vi "ALLARMI_VI.vi"(7 "simulazione":bool, 8 "error in (no error)":errorcluster, 9 "STORICO":refnum<vi>, 10 "STATO SOGLIE IMPOSTATE":refnum<vi>, 11 "Queue Name":string="ALLARMI_Q") -> (0 "error out":errorcluster, 2 "Stopped":bool)   [LabVIEW 2019]
uses:
  TypeDef/cluster allarme cost.ctl
  TypeDef/cluster allarme interp.ctl
  <vilib>/Utility/miscctls.llb/LVRowAndColumnTypeDef.ctl
  <vilib>/Utility/file.llb/Write To Spreadsheet File (string).vi
panel:
  in  "Percorso salvataggio":path
  in  "SALVA STORICO ALLARMI":bool
  out "Array soglie interpolate out":T1[](array[typedef])
  out "Array soglie costanti out":T2[](array[typedef]) caption="STORICO ALLARMI"
  out "DATA OUT":cluster{T2[], T1[]} caption="SITUAZIONE ATTUALE ALLARMI"
  out "elements in queue":i32
  out "STATO":string
  out "LOOP TIME (ms)":u32
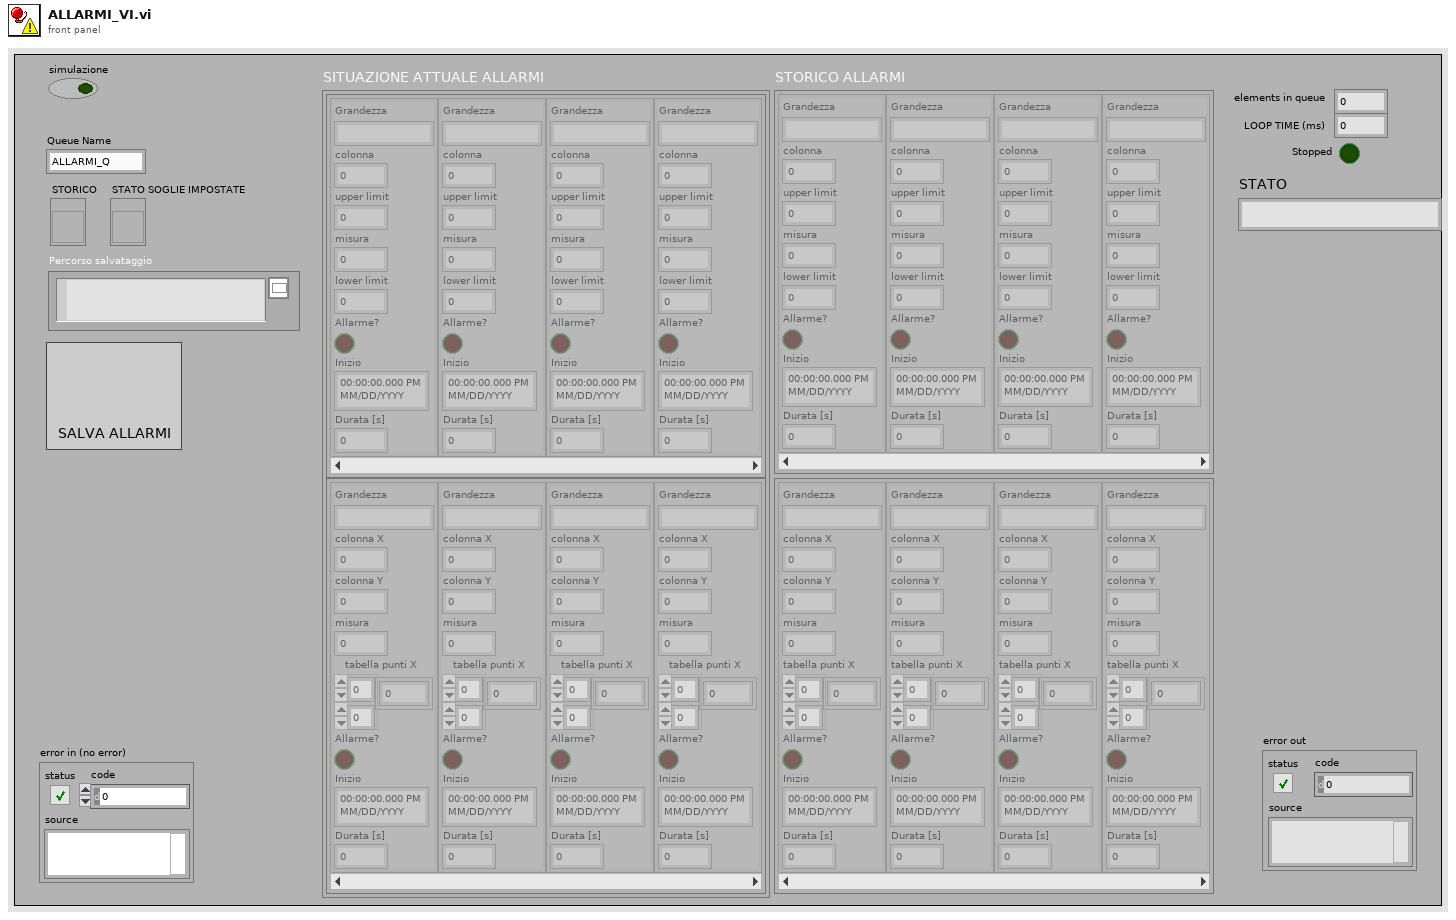
[diagram p1: front panel]
types:
  T1 = typedef "cluster allarme interp.ctl" = cluster{"Grandezza":string, "colonna X":i32, "colonna Y":i32, "misura":dbl, "tabella punti X":dbl[][], "Allarme?":bool, "Inizio":timestamp, "Durata [s]":dbl}
  T2 = typedef "cluster allarme cost.ctl" = cluster{"Grandezza":string, "colonna":i32, "upper limit":dbl, "misura":dbl, "lower limit":dbl, "Allarme?":bool, "Inizio":timestamp, "Durata [s]":dbl}
  T3 = typedef "LVRowAndColumnTypeDef.ctl" = cluster{"Row":i32, "Column":i32}
  T4 = cluster{"Array soglie costanti":T2[], "Array soglie interpolate":T1[]}
  T5 = cluster{"Array of elements":cluster{"String":string, "variant":variant}[], "Single element":cluster{"String":string, "variant":variant}, "enque at\nopposite end (F)":bool, "no replications (F)":bool}
  T6 = enum32{"Invalid", "Standard", "Closed", "Hidden", "Minimized", "Maximized"}
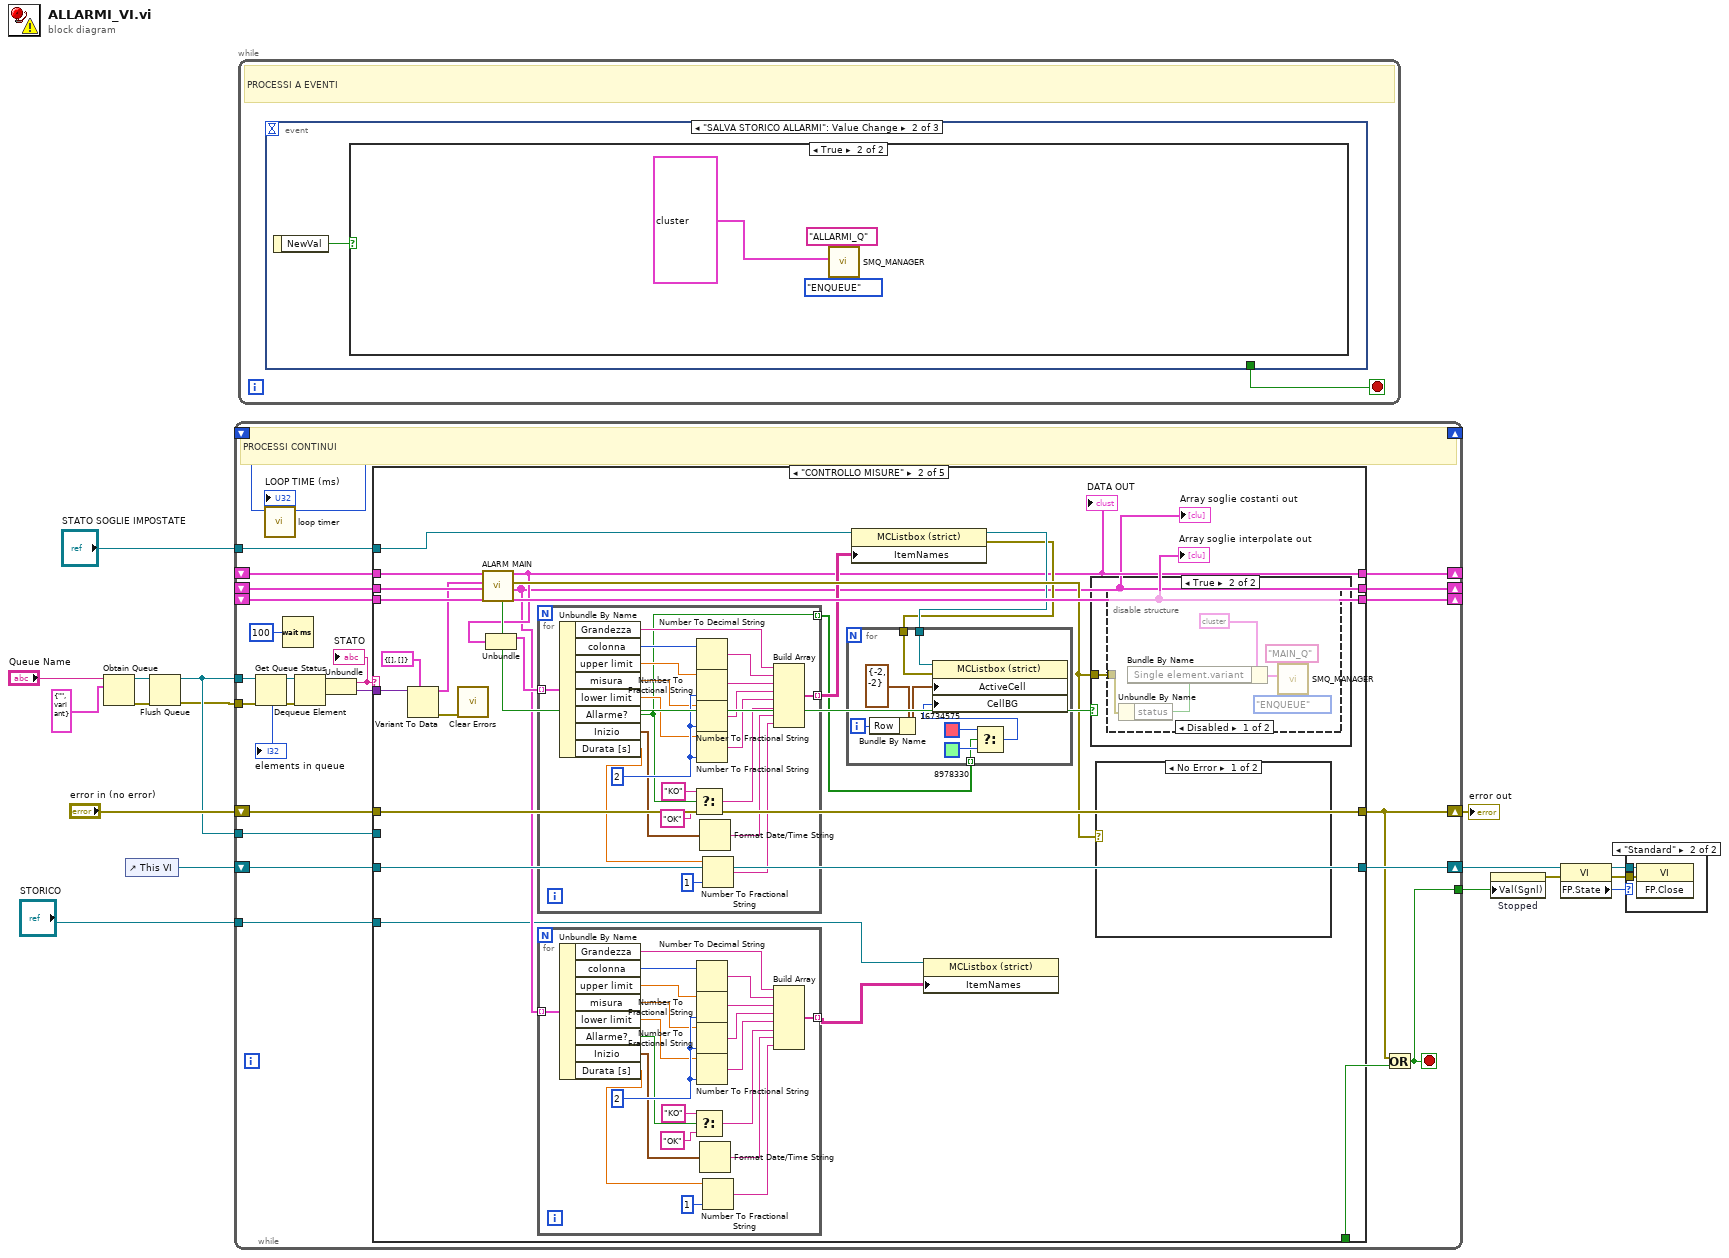
[diagram p0: block diagram]
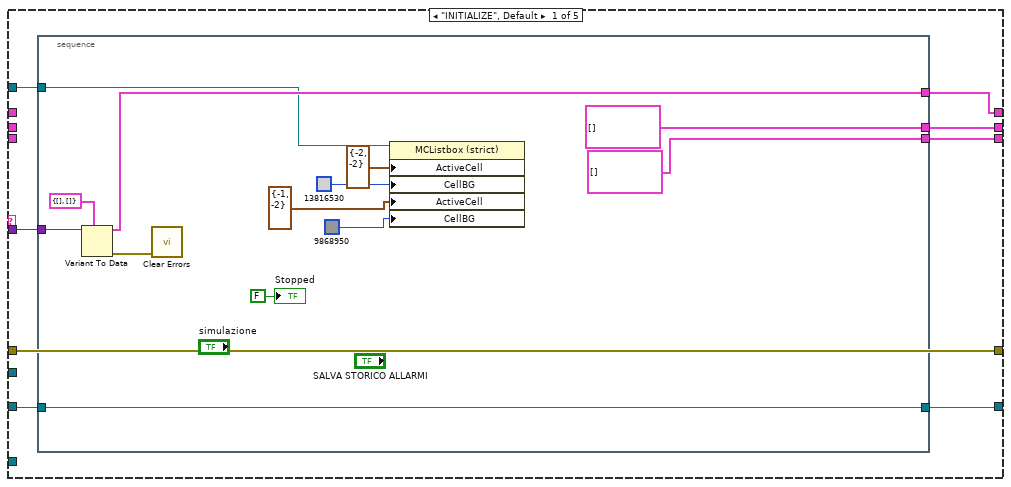
[diagram p3: hidden frame]
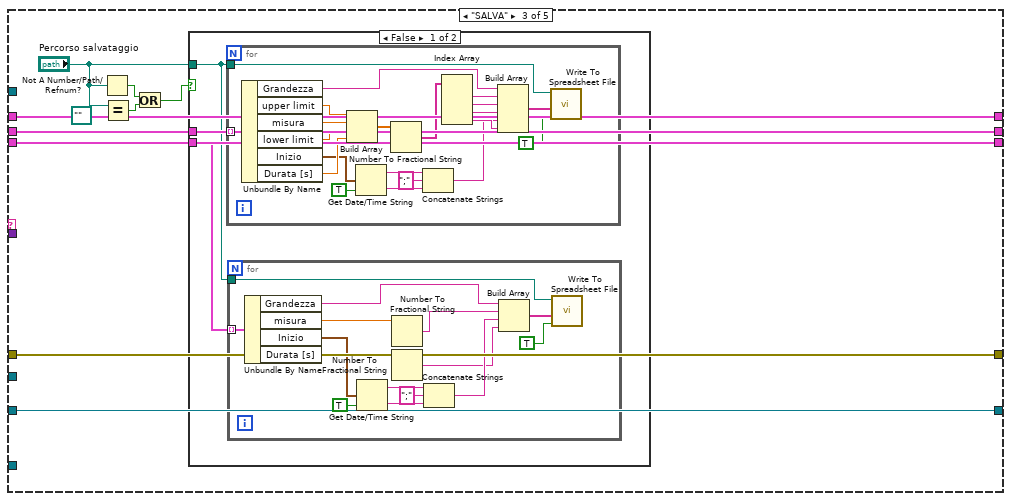
[diagram p7: hidden frame]
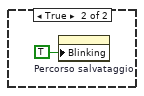
[diagram p8: hidden frame]
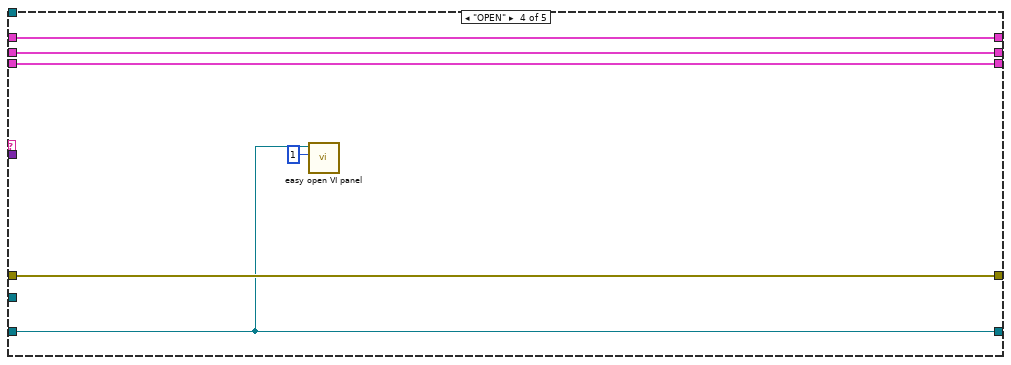
[diagram p9: hidden frame]
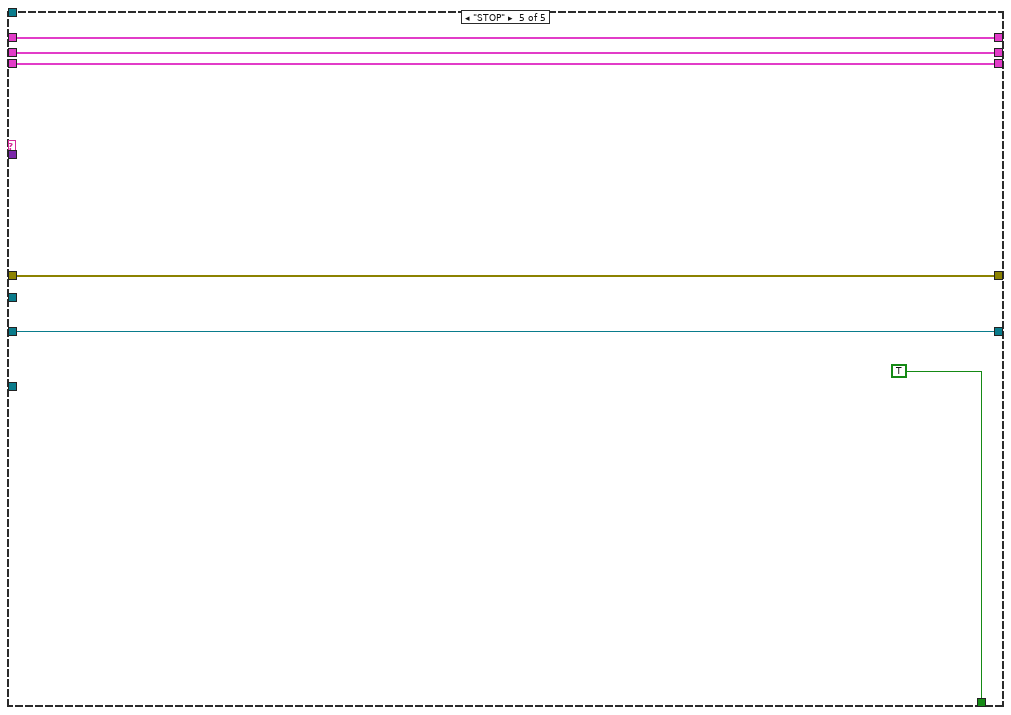
[diagram p10: hidden frame]
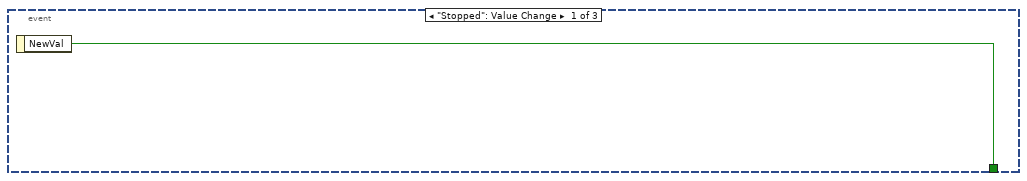
[diagram p11: hidden frame]
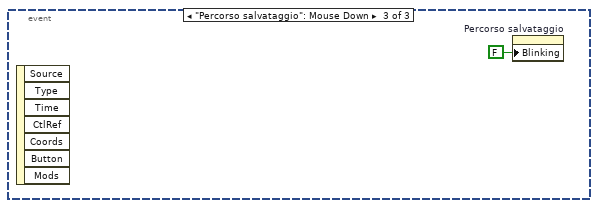
[diagram p13: hidden frame]
diagram:
  n1 = Obtain Queue(name (unnamed)="Queue Name", element data type=cluster{"String":string, "variant":variant} {"String"="", "variant"=variant} ("element")) -> (queue out=w7:refnum<queue>, error out=w6:errorcluster)  [unwired: 3 in, 1 out]
  n2 = control-ref of="This VI"() -> (w3:refnum<vi>)
  n3 = Flush Queue(queue=w7, error in (no error)=w6) -> (queue out=w5:refnum<queue>, error out=w4:errorcluster)  [unwired: 1 out]
  n4 = while {
    shift-right: [w44] -> _
    shift-left: _ -> [w43]
    shift-right: [w41] -> w10
    shift-left: w3 -> [w40]
    shift-right: [w37] -> w13
    shift-left: "error in (no error)" -> [w39]
    tunnel: w5 -> [w31]
    tunnel: w4 -> [w30]
    tunnel: [w34] -> w14
    tunnel: w5 -> [w32]
    shift-right: [w25] -> _
    shift-left: _ -> [w24]
    shift-right: [w23] -> _
    shift-left: _ -> [w22]
    shift-right: [w21] -> _
    shift-left: _ -> [w20]
    tunnel: "STATO SOGLIE IMPOSTATE" -> [w19]
    tunnel: "STORICO" -> [w18]
    stop <- w34 stop-if-true
    # "PROCESSI CONTINUI"
    n5 = Get Queue Status(queue=w31, error in (no error)=w30) -> (queue out=w28:refnum<queue>, error out=w29:errorcluster, # elements in queue=→"elements in queue":i32)  [unwired: 1 in, 5 out]
    n6 = call <userlib>:"loop timer.vi"("millisecond timer IN"=w43) -> ("millisecond timer OUT"=w44:u32, "LOOP TIME (ms)"=→"LOOP TIME (ms)":u32)  [unwired: 9 in]
    n7 = Wait (ms)(milliseconds to wait=u32 100) -> ()  [unwired: 1 out]
    n8 = Dequeue Element(queue=w28, error in (no error)=w29) -> (element=w36:cluster{"String":string, "variant":variant})  [unwired: 1 in, 3 out]
    n9 = Unbundle(w36) -> ("String"=w33:string, "variant"=w35:variant)
    "STATO" <- w33
    n10 = case shown="\"CONTROLLO MISURE\"" w33 {
      tunnel: [_ _ _ _ TRUE] -> w38
      tunnel: [w52 w87 w155 w200 w206] -> w41
      tunnel: w40 -> [w46 w87 w155 w200 w206]
      tunnel: w39 -> [w51 w86 w154 w201 w205]
      tunnel: [w51 w86 w154 w201 w205] -> w37
      tunnel: w35 -> [w49 w85 _ _ _]
      tunnel: w32 -> [_ _ _ _ _]
      tunnel: [w50 w70 w153 w199 w204] -> w25
      tunnel: w24 -> [_ w78 w153 w199 w204]
      tunnel: [w48 w68 w152 w198 w203] -> w23
      tunnel: w22 -> [_ w83 w152 w198 w203]
      tunnel: [w47 w81 w151 w197 w202] -> w21
      tunnel: w20 -> [_ w82 w151 w197 w202]
      tunnel: w19 -> [w45 w74 _ _ _]
      tunnel: w18 -> [_ w67 _ _ _]
      frame "INITIALIZE", Default {
        n11 = stacked-sequence {
          tunnel: [w59] -> w52
          tunnel: [w62] -> w50
          tunnel: w49 -> [w64]
          tunnel: [T2[] [] ("Array soglie costanti")] -> w48
          tunnel: [T1[] [] ("Array soglie interpolate")] -> w47
          tunnel: w46 -> [w59]
          tunnel: w45 -> [w57]
          frame #0 {
            n12 = Variant To Data(type=T4 {"Array soglie costanti"=[], "Array soglie interpolate"=[]} ("data"), Variant=w64) -> (data=w62:T4, error out=w58:errorcluster)  [unwired: 1 in]
            n13 = call <vilib>:"Clear Errors.vi"("error in (no error)"=w58) -> ()  [unwired: 5 in, 2 out]
            n14 = property class="MCListbox (strict)"(reference=w57, "ActiveCell"=T3 {"Row"=-2, "Column"=-2} ("Active Cell:Active Cell"), "CellBG"=u32 13816530, "ActiveCell"=T3 {"Row"=-1, "Column"=-2} ("Active Cell:Active Cell"), "CellBG"=u32 9868950) -> ()  [unwired: 1 in, 2 out]
            "Stopped" <- FALSE ("Stop")
          }
        }
      }
      frame "CONTROLLO MISURE" {
        n15 = Variant To Data(type=T4 {"Array soglie costanti"=[], "Array soglie interpolate"=[]}, Variant=w85) -> (data=w79:T4, error out=w76:errorcluster)  [unwired: 1 in]
        n16 = call <vilib>:"Clear Errors.vi"("error in (no error)"=w76) -> ()  [unwired: 5 in, 2 out]
        n17 = call "ALARM MAIN.vi"("Array soglie interpolate in"=w82, "Array soglie costanti in"=w83, "new data"=w79, "old data"=w78) -> ("Array soglie interpolate out"=w81:T1[], "Array soglie costanti out"=w68:T2[], "alarm error"=w77:errorcluster, "DATA OUT"=w70:cluster{T2[], T1[]}, "AGGIORNA?"=w80:bool)  [unwired: 3 in]
        "DATA OUT" <- w70
        "Array soglie costanti out" <- w68
        "Array soglie interpolate out" <- w81
        n18 = Unbundle(w70) -> (w69:T2[])  [unwired: 1 out]
        n19 = for {
          tunnel: w69 -> [w138] mode=indexing
          tunnel: [w120] -> w75 mode=indexing
          tunnel: [w118] -> w71 mode=indexing
          w135 = i16 2 ("precision (6)")
          n20 = Unbundle By Name(w138) -> ("Grandezza"=w119:string, "colonna"=w137:i32, "upper limit"=w136:dbl, "misura"=w134:dbl, "lower limit"=w133:dbl, "Allarme?"=w118:bool, "Inizio"=w130:timestamp, "Durata [s]"=w129:dbl)
          n21 = Select(t="KO", s=w118, f="OK") -> (s? t:f=w123:string)
          n22 = Number To Decimal String(number=w137) -> (decimal integer string=w127:string)  [unwired: 1 in]
          n23 = Number To Fractional String(number=w136, precision (6)=w135) -> (F-format string=w126:string)  [unwired: 2 in]
          n24 = Number To Fractional String(number=w134, precision (6)=w135) -> (F-format string=w125:string)  [unwired: 2 in]
          n25 = Number To Fractional String(number=w133, precision (6)=w135) -> (F-format string=w124:string)  [unwired: 2 in]
          n26 = Format Date/Time String(seconds (now)=w130) -> (date/time string=w122:string)  [unwired: 2 in]
          n27 = Number To Fractional String(number=w129, precision (6)=i16 1) -> (F-format string=w121:string)  [unwired: 2 in]
          n28 = Build Array(w119, w127, w126, w125, w124, w123, w122, w121) -> (w120:string[])
        }
        n29 = for {
          tunnel: w68 -> [w108] mode=indexing
          tunnel: [w90] -> w66 mode=indexing
          w105 = i16 2 ("precision (6)")
          n30 = Unbundle By Name(w108) -> ("Grandezza"=w89:string, "colonna"=w107:i32, "upper limit"=w106:dbl, "misura"=w104:dbl, "lower limit"=w103:dbl, "Allarme?"=w88:bool, "Inizio"=w100:timestamp, "Durata [s]"=w99:dbl)
          n31 = Select(t="KO", s=w88, f="OK") -> (s? t:f=w93:string)
          n32 = Number To Decimal String(number=w107) -> (decimal integer string=w97:string)  [unwired: 1 in]
          n33 = Number To Fractional String(number=w106, precision (6)=w105) -> (F-format string=w96:string)  [unwired: 2 in]
          n34 = Number To Fractional String(number=w104, precision (6)=w105) -> (F-format string=w95:string)  [unwired: 2 in]
          n35 = Number To Fractional String(number=w103, precision (6)=w105) -> (F-format string=w94:string)  [unwired: 2 in]
          n36 = Format Date/Time String(seconds (now)=w100) -> (date/time string=w92:string)  [unwired: 2 in]
          n37 = Number To Fractional String(number=w99, precision (6)=i16 1) -> (F-format string=w91:string)  [unwired: 2 in]
          n38 = Build Array(w89, w97, w96, w95, w94, w93, w92, w91) -> (w90:string[])
        }
        n39 = property class="MCListbox (strict)"(reference=w74, "ItemNames"=w75) -> (reference out=w73:refnum<vi>, error out=w72:errorcluster)  [unwired: 1 in]
        n40 = for {
          tunnel: w73 -> [w117]
          tunnel: w72 -> [w116]
          tunnel: w71 -> [w110] mode=indexing
          i -> [w114]
          n41 = Bundle By Name(cluster=T3 {"Row"=-2, "Column"=-2} ("Active Cell:Active Cell"), "Row"=w114) -> (w113:T3)
          n42 = Select(t=u32 16734575, s=w110, f=u32 8978330) -> (s? t:f=w109:u32)
          n43 = property class="MCListbox (strict)"(reference=w117, error in=w116, "ActiveCell"=w113, "CellBG"=w109) -> ()  [unwired: 2 out]
        }
        n44 = property class="MCListbox (strict)"(reference=w67, "ItemNames"=w66) -> ()  [unwired: 1 in, 2 out]
        n45 = case shown="True" w80 {
          tunnel: w77 -> [_ w139]
          frame False {
          }
          frame True {
            n46 = disable-structure shown="Disabled" {
              disable-tunnel: w139 -> [w141 _]
              frame Disabled {
                n47 = Unbundle By Name(w141) -> ("status"=w140:bool)
                n48 = Bundle By Name(cluster=T5 {"Array of elements"=[], "Single element"={"String"="ALLARME", "variant"=variant}, "enque at\nopposite end (F)"=FALSE, "no replications (F)"=FALSE} ("Enqueue cluster"), "Single element.variant"=w140) -> (w142:T5)
                n49 = call <userlib>:"SMQ_MANAGER.vi"("Function"=enum16{"INITIALIZE", "ENQUEUE", "STOP ALL"}."ENQUEUE", "Queue name"="MAIN_Q", "Enqueue cluster"=w142) -> ()  [unwired: 8 in, 1 out]
              }
              frame Enabled {
              }
            }
          }
        }
        n50 = case shown="No Error" w77 {
          frame No Error {
          }
          frame Error {
          }
        }
      }
      frame "SALVA" {
        n51 = Not A Number/Path/Refnum?(number/path/refnum="Percorso salvataggio") -> (NaN/Path/Refnum?=w150:bool)
        n52 = Equal?(x="Percorso salvataggio", y=path "") -> (x = y?=w147:bool)
        n53 = Or(x=w150, y=w147) -> (x .or. y?=w146:bool)
        n54 = case shown="False" w146 {
          tunnel: w152 -> [w158 _]
          tunnel: "Percorso salvataggio" -> [w156 _]
          tunnel: w151 -> [w157 _]
          frame False {
            n55 = for {
              tunnel: w158 -> [w194] mode=indexing
              tunnel: w156 -> [w174]
              n56 = Unbundle By Name(w194) -> ("Grandezza"=w184:string, "upper limit"=w193:dbl, "misura"=w192:dbl, "lower limit"=w191:dbl, "Inizio"=w183:timestamp, "Durata [s]"=w190:dbl)
              n57 = Build Array(w193, w192, w191, w190) -> (w189:dbl[])
              n58 = Get Date/Time String(seconds (now)=w183, want seconds? (F)=TRUE) -> (date string=w181:string, time string=w179:string)  [unwired: 1 in]
              n59 = Number To Fractional String(number=w189) -> (F-format string=w188:string[])  [unwired: 3 in]
              n60 = Concatenate Strings(w181, ";" ("string"), w179) -> (w177:string)
              n61 = Index Array(array=w188) -> (element #1=w185:string, element #2=w187:string, element #3=w186:string, element #4=w178:string)  [unwired: 4 in]
              n62 = Build Array(w184, w185, w187, w186, w177, w178) -> (w176:string[])
              n63 = call-poly <vilib>:"Write To Spreadsheet File.vi"("append to file? (new file:F)"=TRUE, "1D data"=w176, "file path (dialog if empty)"=w174) -> ()  [unwired: 5 in, 1 out]
            }
            n64 = for {
              tunnel: w157 -> [w173] mode=indexing
              tunnel: w156 -> [w163]
              n65 = Unbundle By Name(w173) -> ("Grandezza"=w172:string, "misura"=w162:dbl, "Inizio"=w171:timestamp, "Durata [s]"=w160:dbl)
              n66 = Get Date/Time String(seconds (now)=w171, want seconds? (F)=TRUE) -> (date string=w169:string, time string=w167:string)  [unwired: 1 in]
              n67 = Number To Fractional String(number=w162) -> (F-format string=w161:string)  [unwired: 3 in]
              n68 = Number To Fractional String(number=w160) -> (F-format string=w159:string)  [unwired: 3 in]
              n69 = Concatenate Strings(w169, ";" ("string"), w167) -> (w166:string)
              n70 = Build Array(w172, w161, w166, w159) -> (w165:string[])
              n71 = call-poly <vilib>:"Write To Spreadsheet File.vi"("append to file? (new file:F)"=TRUE, "1D data"=w165, "file path (dialog if empty)"=w163) -> ()  [unwired: 5 in, 1 out]
            }
          }
          frame True {
            n72 = property on="Percorso salvataggio" class="Path"("Blinking"=TRUE) -> ()  [unwired: 2 in, 2 out]
          }
        }
      }
      frame "OPEN" {
        n73 = call <userlib>:"easy open VI panel.vi"("Monitor(1)"=u16 1, "VI in"=w200) -> ()  [unwired: 9 in, 1 out]
      }
      frame "STOP" {
      }
    }
    n74 = Or(x=w37, y=w38) -> (x .or. y?=w34:bool)
  }
  "error out" <- w13
  n75 = while {
    stop <- w208 stop-if-true
    # "PROCESSI A EVENTI"
    n76 = event shown="[1] \"SALVA STORICO ALLARMI\": Value Change" {
      selector: _ -> [_ _ _]
      dyn-events: _ -> [_ _ _]
      timeout: _ -> [_ _ _]
      tunnel: [w209 _ _] -> w208
      event "Stopped": Value Change {
        n77 = event-data() -> ("NewVal"=w209:bool)  [unwired: 1 in]
      }
      event "SALVA STORICO ALLARMI": Value Change {
        n78 = event-data() -> ("NewVal"=w210:bool)  [unwired: 1 in]
        n79 = case shown="True" w210 {
          frame False {
          }
          frame True {
            n80 = call <userlib>:"SMQ_MANAGER.vi"("Function"=enum16{"INITIALIZE", "ENQUEUE", "STOP ALL"}."ENQUEUE", "Queue name"="ALLARMI_Q", "Enqueue cluster"=T5 {"Array of elements"=[], "Single element"={"String"="SALVA", "variant"=variant}, "enque at\nopposite end (F)"=FALSE, "no replications (F)"=FALSE}) -> ()  [unwired: 8 in, 1 out]
          }
        }
      }
      event "Percorso salvataggio": Mouse Down {
        n81 = event-data() -> ()  [unwired: 1 in, 7 out]
        n82 = property on="Percorso salvataggio" class="Path"("Blinking"=FALSE) -> ()  [unwired: 2 in, 2 out]
      }
    }
  }
  n83 = property on="Stopped" class="Bool (strict)"("Val(Sgnl)"=w14) -> (error out=w9:errorcluster)  [unwired: 2 in, 1 out]
  n84 = property class="VI"(reference=w10, error in=w9) -> (reference out=w12:refnum<vi>, error out=w8:errorcluster, "FP.State"=w11:T6)
  n85 = case shown="\"Standard\"" w11 {
    tunnel: w12 -> [_ w216]
    tunnel: w8 -> [_ w215]
    frame "Invalid", Default {
    }
    frame "Standard" {
      n86 = invoke class="VI" method="FP.Close"(reference=w216, error in=w215) -> ()  [unwired: 1 in, 3 out]
    }
  }
